vi "Poll.FormatErrorStatus.vi"(5 "Read Table":variant, 7 "Write Table":variant, 8 "error in (no error)":errorcluster, 9 "Read Code":i32, 10 "Write Code":i32, 11 "TotalTags":u32) -> (0 "error out":errorcluster, 3 "ErrorStatus":u32[](array[numeric]))   [LabVIEW 2015, in "OPC UA Client Engine.lvlib"]
uses:
  OPC UA Client Engine.lvlib
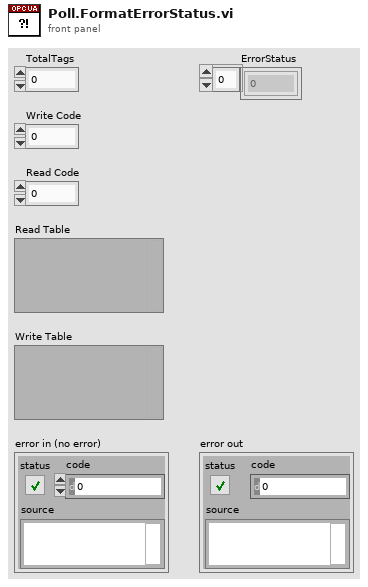
[diagram p1: front panel]
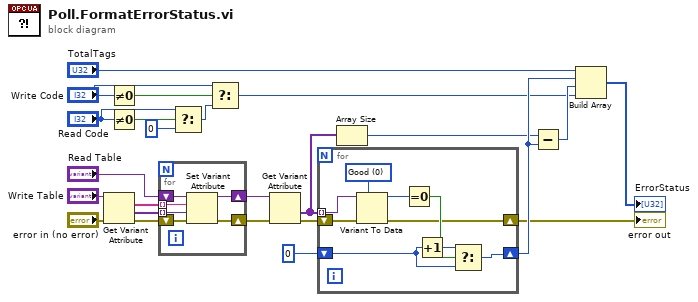
[diagram p0: block diagram]
diagram:
  n1 = Get Variant Attribute(Variant="Write Table", error in="error in (no error)") -> (names=w2:string[], values=w3:variant[], error out=w4:errorcluster)  [unwired: 2 in, 1 out]
  n2 = Not Equal To 0?(x="Write Code") -> (x != 0?=w11:bool)
  n3 = Not Equal To 0?(x="Read Code") -> (x != 0?=w15:bool)
  n4 = for {
    tunnel: w2 -> [w30] mode=indexing
    tunnel: w3 -> [w29] mode=indexing
    shift-right: [w27] -> w5
    shift-left: "Read Table" -> [w28]
    shift-right: [w25] -> w6
    shift-left: w4 -> [w26]
    n5 = Set Variant Attribute(Variant=w28, name=w30, value=w29, error in=w26) -> (Variant out=w27:variant, error out=w25:errorcluster)  [unwired: 1 out]
  }
  n6 = Select(t="Read Code", s=w15, f=0) -> (s? t:f=w13:i32)
  n7 = Select(t="Write Code", s=w11, f=w13) -> (s? t:f=w17:i32)
  n8 = Get Variant Attribute(Variant=w5, error in=w6) -> (values=w9:variant[], error out=w7:errorcluster)  [unwired: 2 in, 2 out]
  n9 = for {
    tunnel: w9 -> [w37] mode=indexing
    shift-right: [w32] -> w22
    shift-left: 0 -> [w34]
    shift-right: [w31] -> w18
    shift-left: w7 -> [w39]
    w38 = u32 0 items=["Good"=0, "Bad_AttributeIdInvalid"=2153906176, "Bad_BrowseDirectionInvalid"=2152529920, "Bad_BrowseNameInvalid"=2153775104, "Bad_ContentFilterInvalid"=2152202240, "Bad_ContinuationPointInvalid"=2152333312, "Bad_DataEncodingInvalid"=2151153664, "Bad_DataEncodingUnsupported"=2151219200, "Bad_EventFilterInvalid"=2152136704, "Bad_FilterNotAllowed"=2152005632, "Bad_FilterOperandInvalid"=2160132096, "Bad_HistoryOperationInvalid"=2154889216, "Bad_HistoryOperationUnsupported"=2154954752, "Bad_IndexRangeInvalid"=2151022592, "Bad_IndexRangeNoData"=2151088128, "Bad_MonitoredItemFilterInvalid"=2151874560, "Bad_MonitoredItemFilterUnsupported"=2151940096, "Bad_MonitoredItemIdInvalid"=2151809024, "Bad_MonitoringModeInvalid"=2151743488, "Bad_NoCommunication"=2150694912, "Bad_NoContinuationPoints"=2152398848, "Bad_NodeClassInvalid"=2153709568, "Bad_NodeIdInvalid"=2150825984, "Bad_NodeIdUnknown"=2150891520, "Bad_NoDeleteRights"=2154364928, "Bad_NodeNotInView"=2152595456, "Bad_NotFound"=2151546880, "Bad_NotImplemented"=2151677952, "Bad_NotReadable"=2151284736, "Bad_NotSupported"=2151481344, "Bad_NotWritable"=2151350272, "Bad_ObjectDeleted"=2151612416, "Bad_OutOfRange"=2151415808, "Bad_ReferenceTypeIdInvalid"=2152464384, "Bad_SourceNodeIdInvalid"=2154037248, "Bad_StructureMissing"=2152071168, "Bad_TargetNodeIdInvalid"=2154102784, "Bad_TypeDefinitionInvalid"=2153971712, "Bad_TypeMismatch"=2155085824, "Bad_WaitingForInitialData"=2150760448] ("status")
    n10 = Variant To Data(error in=w39, type=w38, Variant=w37) -> (data=w36:u32, error out=w31:errorcluster)
    n11 = Equal To 0?(x=w36) -> (x = 0?=w35:bool)
    n12 = Increment(x=w34) -> (x+1=w33:i32)
    n13 = Select(t=w33, s=w35, f=w34) -> (s? t:f=w32:i32)
  }
  "error out" <- w18
  n14 = Array Size(array=w9) -> (size(s)=w10:i32)
  n15 = Subtract(x=w10, y=w22) -> (x-y=w23:i32)
  n16 = Build Array("TotalTags", w22, w23, w17) -> (→"ErrorStatus":u32[])
